vi "T7 Stream Globals KAG.vi"() -> ()   [LabVIEW 2015]
doc: "T7 Stream Global Controls"
panel:
  in  "Device IP":string="192.168.126.147"
  in  "Allow Checksum Errors":bool=TRUE
  out "Calibration Constants":T1(array[cluster]) {"PSlope" format="%#.13f"; "NSlope" format="%#.13f"; "AvgSlope" format="%#.13f"; "Center" format="%#.13f"; "Offset" format="%#.13f"}
  out "error out":errorcluster
  out "Packet Counter Out":i32
  in  "Connection ID Out":refnum<k5>
  in  "Scan Table":T2(array[cluster])=[{"Channel"=0, "BipGain"=0, "Input Config"="Single-Ended"}, {"Channel"=2, "BipGain"=0, "Input Config"="Single-Ended"}, {"Channel"=4, "BipGain"=0, "Input Config"="Single-Ended"}, {"Channel"=6, "BipGain"=0, "Input Config"="Single-Ended"}] {"BipGain" max=3 step=1; "Channel" step=1}
  # "Gain"
  # "x1"
  # "x10"
  # "x100"
  # "x1000"
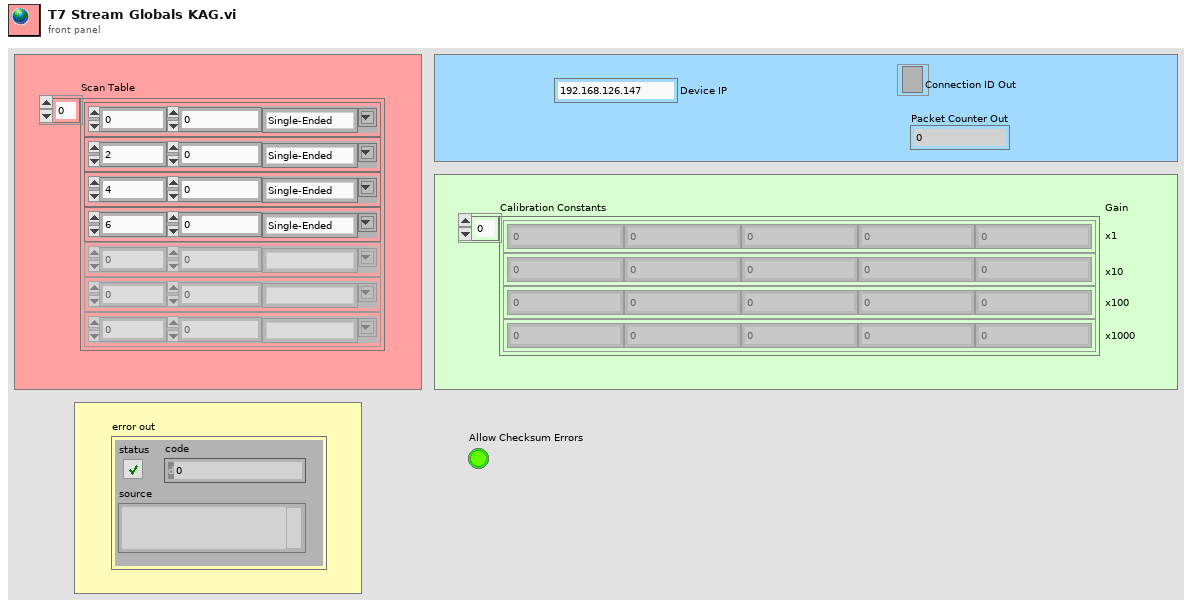
[diagram p1: front panel]
types:
  T1 = cluster{"PSlope":dbl, "NSlope":dbl, "AvgSlope":dbl, "Center":dbl, "Offset":dbl}[]
  T2 = cluster{"Channel":u32, "BipGain":u32, "Input Config":string}[]
diagram:
